vi "Ejemplo.vi"() -> ()   [LabVIEW 2020]
panel:
  in  "Tabla":string[][](table) caption="Result Set (from first statement with results)"
  in  "Multicolumn Listbox":i32(listbox)
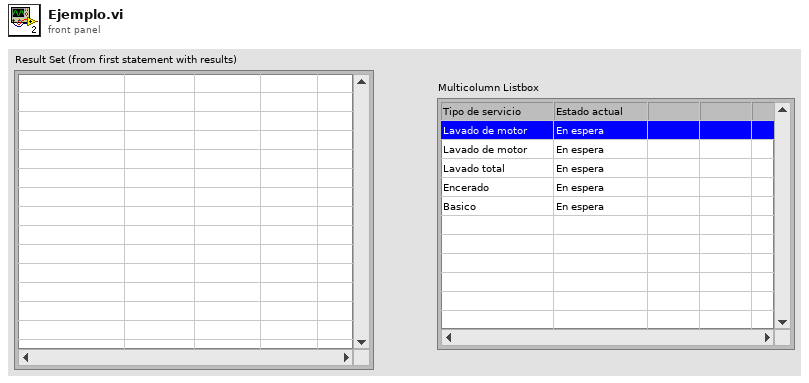
[diagram p1: front panel]
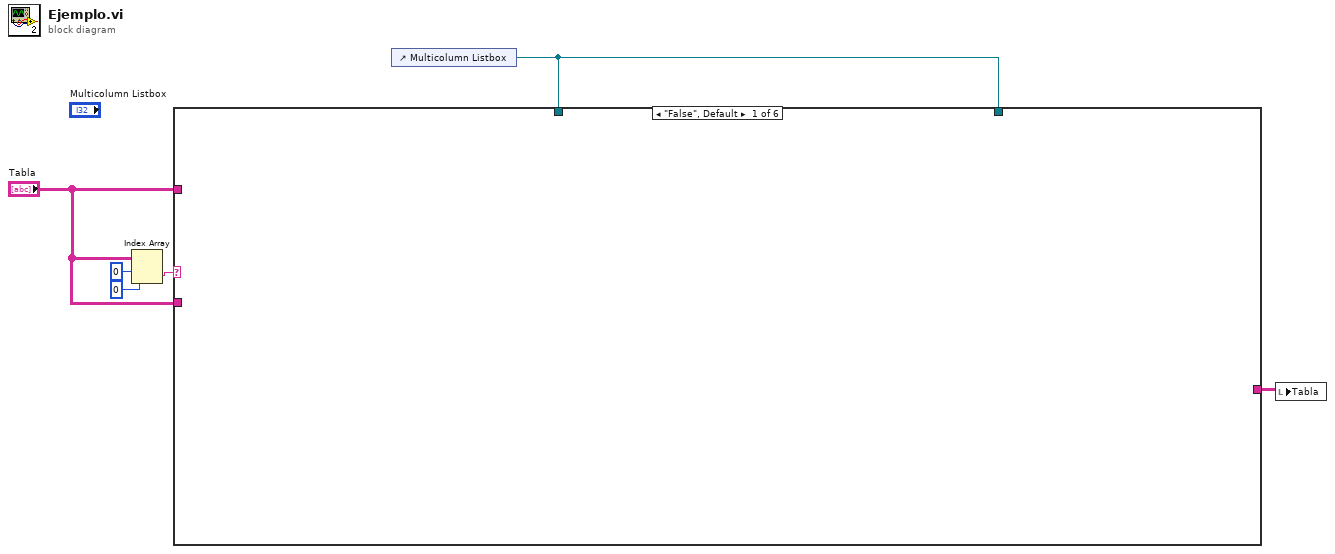
[diagram p0: block diagram]
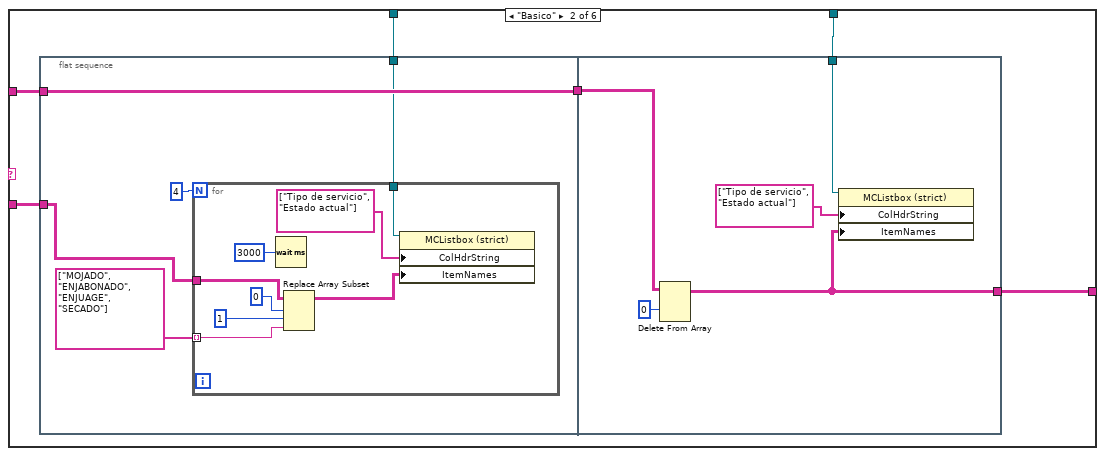
[diagram p2: hidden frame]
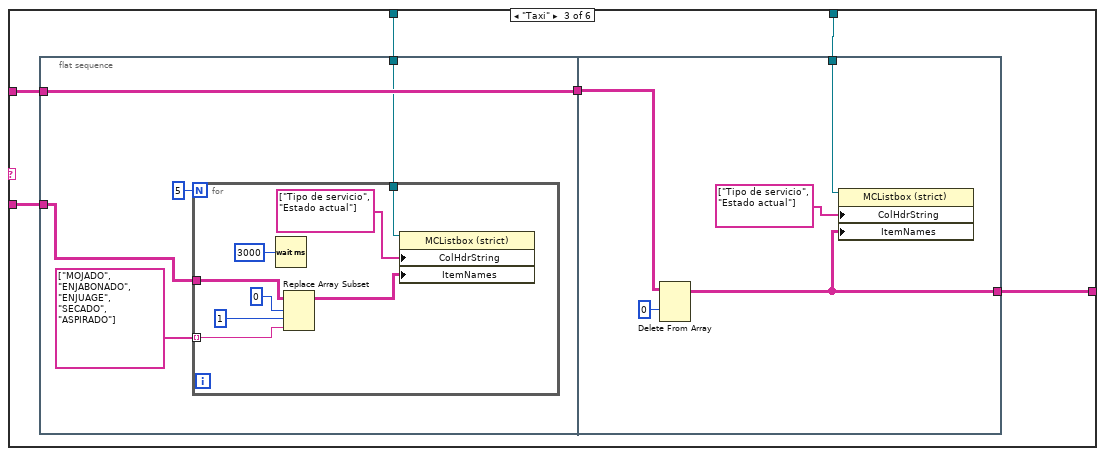
[diagram p3: hidden frame]
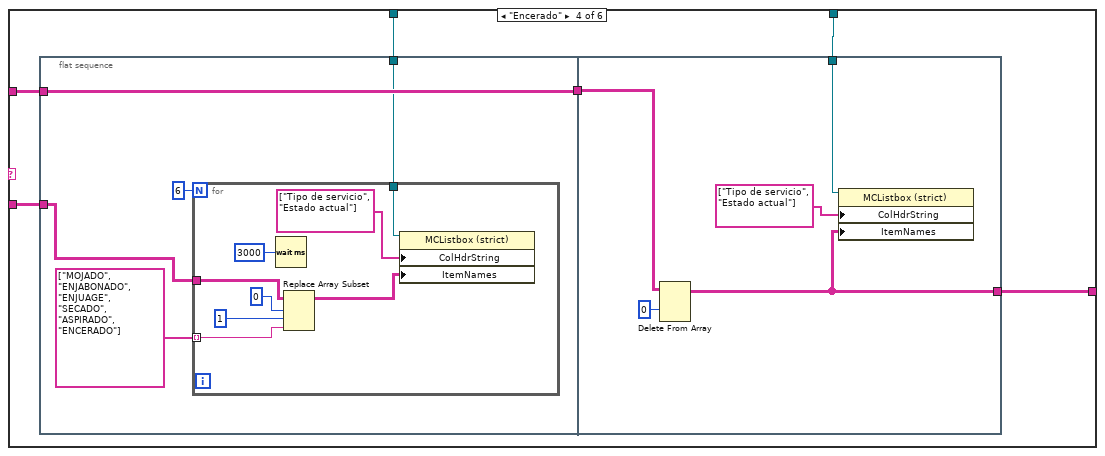
[diagram p4: hidden frame]
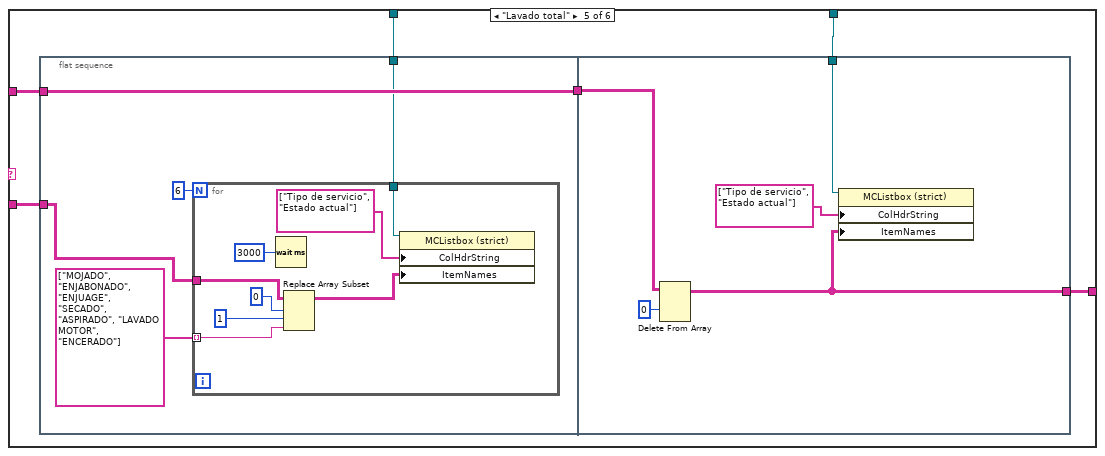
[diagram p5: hidden frame]
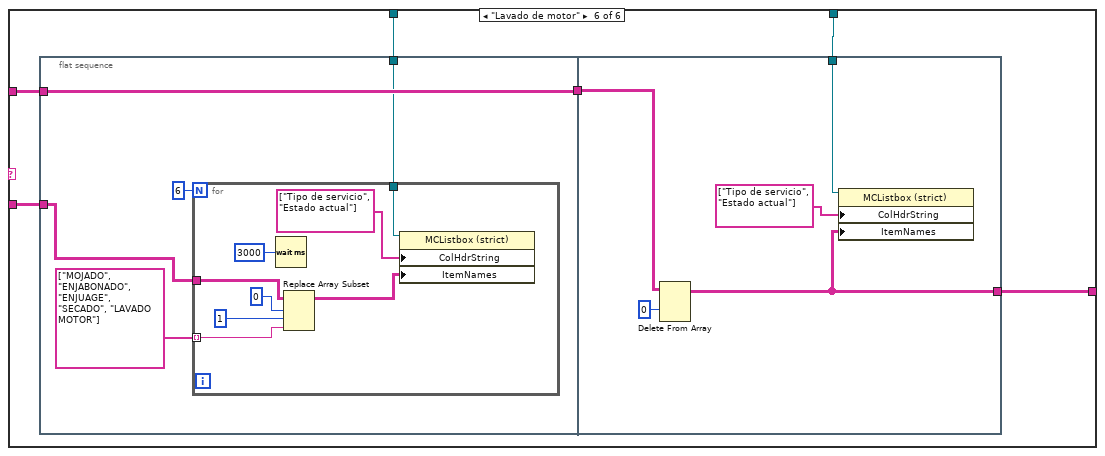
[diagram p6: hidden frame]
diagram:
  n1 = Index Array(array="Tabla", index (row)=0 ("index"), index (col)=0 ("disabled index (col)")) -> (element=w4:string)
  n2 = control-ref of="Multicolumn Listbox"() -> (w3:refnum<vi>)
  n3 = case shown="\"False\", Default" w4 {
    tunnel: "Tabla" -> [_ w12 w36 w60 w84 w108]
    tunnel: "Tabla" -> [_ w11 w35 w59 w83 w107]
    tunnel: w3 -> [_ w9 w33 w57 w81 w105]
    tunnel: w3 -> [_ w8 w32 w56 w80 w104]
    tunnel: [_ w7 w31 w55 w79 w103] -> w1
    frame "False", Default {
    }
    frame "Basico" {
      n4 = flat-sequence {
        tunnel: w12 -> [w15]
        tunnel: w11 -> [w14]
        tunnel: [w14] -> w10
        tunnel: w8 -> [w13]
        tunnel: w10 -> [w28]
        tunnel: w9 -> [w30]
        tunnel: [w26] -> w7
        frame #0 {
          n5 = for {
            N: 4 -> [_]
            tunnel: w15 -> [w25]
            tunnel: string[] ["MOJADO", "ENJABONADO", "ENJUAGE", "SECADO"] -> [w22] mode=indexing
            tunnel: w13 -> [w18]
            n6 = Wait (ms)(milliseconds to wait=u32 3000) -> ()  [unwired: 1 out]
            n7 = Replace Array Subset(array=w25, new element=w22, index (row)=0, index (col)=1 ("disabled index (col)")) -> (w19:string[][])
            n8 = property on="Property Node" class="MCListbox (strict)"(reference=w18, "ColHdrString"=string[] ["Tipo de servicio", "Estado actual"] ("Column Header Strings[]"), "ItemNames"=w19) -> ()  [unwired: 1 in, 2 out]
          }
        }
        frame #1 {
          n9 = Delete From Array(array=w28, index (row)=0) -> (array with subset deleted=w26:string[][])  [unwired: 2 in, 1 out]
          n10 = property on="Property Node" class="MCListbox (strict)"(reference=w30, "ColHdrString"=string[] ["Tipo de servicio", "Estado actual"] ("Column Header Strings[]"), "ItemNames"=w26) -> ()  [unwired: 1 in, 2 out]
        }
      }
    }
    frame "Taxi" {
      n11 = flat-sequence {
        tunnel: w36 -> [w39]
        tunnel: w35 -> [w38]
        tunnel: [w38] -> w34
        tunnel: w32 -> [w37]
        tunnel: w34 -> [w52]
        tunnel: w33 -> [w54]
        tunnel: [w50] -> w31
        frame #0 {
          n12 = for {
            N: 5 -> [_]
            tunnel: w39 -> [w49]
            tunnel: string[] ["MOJADO", "ENJABONADO", "ENJUAGE", "SECADO", "ASPIRADO"] -> [w46] mode=indexing
            tunnel: w37 -> [w42]
            n13 = Wait (ms)(milliseconds to wait=u32 3000) -> ()  [unwired: 1 out]
            n14 = Replace Array Subset(array=w49, new element=w46, index (row)=0, index (col)=1 ("disabled index (col)")) -> (w43:string[][])
            n15 = property on="Property Node" class="MCListbox (strict)"(reference=w42, "ColHdrString"=string[] ["Tipo de servicio", "Estado actual"] ("Column Header Strings[]"), "ItemNames"=w43) -> ()  [unwired: 1 in, 2 out]
          }
        }
        frame #1 {
          n16 = Delete From Array(array=w52, index (row)=0) -> (array with subset deleted=w50:string[][])  [unwired: 2 in, 1 out]
          n17 = property on="Property Node" class="MCListbox (strict)"(reference=w54, "ColHdrString"=string[] ["Tipo de servicio", "Estado actual"] ("Column Header Strings[]"), "ItemNames"=w50) -> ()  [unwired: 1 in, 2 out]
        }
      }
    }
    frame "Encerado" {
      n18 = flat-sequence {
        tunnel: w60 -> [w63]
        tunnel: w59 -> [w62]
        tunnel: [w62] -> w58
        tunnel: w56 -> [w61]
        tunnel: w58 -> [w76]
        tunnel: w57 -> [w78]
        tunnel: [w74] -> w55
        frame #0 {
          n19 = for {
            N: 6 -> [_]
            tunnel: w63 -> [w73]
            tunnel: string[] ["MOJADO", "ENJABONADO", "ENJUAGE", "SECADO", "ASPIRADO", "ENCERADO"] -> [w70] mode=indexing
            tunnel: w61 -> [w66]
            n20 = Wait (ms)(milliseconds to wait=u32 3000) -> ()  [unwired: 1 out]
            n21 = Replace Array Subset(array=w73, new element=w70, index (row)=0, index (col)=1 ("disabled index (col)")) -> (w67:string[][])
            n22 = property on="Property Node" class="MCListbox (strict)"(reference=w66, "ColHdrString"=string[] ["Tipo de servicio", "Estado actual"] ("Column Header Strings[]"), "ItemNames"=w67) -> ()  [unwired: 1 in, 2 out]
          }
        }
        frame #1 {
          n23 = Delete From Array(array=w76, index (row)=0) -> (array with subset deleted=w74:string[][])  [unwired: 2 in, 1 out]
          n24 = property on="Property Node" class="MCListbox (strict)"(reference=w78, "ColHdrString"=string[] ["Tipo de servicio", "Estado actual"] ("Column Header Strings[]"), "ItemNames"=w74) -> ()  [unwired: 1 in, 2 out]
        }
      }
    }
    frame "Lavado total" {
      n25 = flat-sequence {
        tunnel: w84 -> [w87]
        tunnel: w83 -> [w86]
        tunnel: [w86] -> w82
        tunnel: w80 -> [w85]
        tunnel: w82 -> [w100]
        tunnel: w81 -> [w102]
        tunnel: [w98] -> w79
        frame #0 {
          n26 = for {
            N: 6 -> [_]
            tunnel: w87 -> [w97]
            tunnel: string[] ["MOJADO", "ENJABONADO", "ENJUAGE", "SECADO", "ASPIRADO", "LAVADO MOTOR", "ENCERADO"] -> [w94] mode=indexing
            tunnel: w85 -> [w90]
            n27 = Wait (ms)(milliseconds to wait=u32 3000) -> ()  [unwired: 1 out]
            n28 = Replace Array Subset(array=w97, new element=w94, index (row)=0, index (col)=1 ("disabled index (col)")) -> (w91:string[][])
            n29 = property on="Property Node" class="MCListbox (strict)"(reference=w90, "ColHdrString"=string[] ["Tipo de servicio", "Estado actual"] ("Column Header Strings[]"), "ItemNames"=w91) -> ()  [unwired: 1 in, 2 out]
          }
        }
        frame #1 {
          n30 = Delete From Array(array=w100, index (row)=0) -> (array with subset deleted=w98:string[][])  [unwired: 2 in, 1 out]
          n31 = property on="Property Node" class="MCListbox (strict)"(reference=w102, "ColHdrString"=string[] ["Tipo de servicio", "Estado actual"] ("Column Header Strings[]"), "ItemNames"=w98) -> ()  [unwired: 1 in, 2 out]
        }
      }
    }
    frame "Lavado de motor" {
      n32 = flat-sequence {
        tunnel: w108 -> [w111]
        tunnel: w107 -> [w110]
        tunnel: [w110] -> w106
        tunnel: w104 -> [w109]
        tunnel: w106 -> [w124]
        tunnel: w105 -> [w126]
        tunnel: [w122] -> w103
        frame #0 {
          n33 = for {
            N: 6 -> [_]
            tunnel: w111 -> [w121]
            tunnel: string[] ["MOJADO", "ENJABONADO", "ENJUAGE", "SECADO", "LAVADO MOTOR"] -> [w118] mode=indexing
            tunnel: w109 -> [w114]
            n34 = Wait (ms)(milliseconds to wait=u32 3000) -> ()  [unwired: 1 out]
            n35 = Replace Array Subset(array=w121, new element=w118, index (row)=0, index (col)=1 ("disabled index (col)")) -> (w115:string[][])
            n36 = property on="Property Node" class="MCListbox (strict)"(reference=w114, "ColHdrString"=string[] ["Tipo de servicio", "Estado actual"] ("Column Header Strings[]"), "ItemNames"=w115) -> ()  [unwired: 1 in, 2 out]
          }
        }
        frame #1 {
          n37 = Delete From Array(array=w124, index (row)=0) -> (array with subset deleted=w122:string[][])  [unwired: 2 in, 1 out]
          n38 = property on="Property Node" class="MCListbox (strict)"(reference=w126, "ColHdrString"=string[] ["Tipo de servicio", "Estado actual"] ("Column Header Strings[]"), "ItemNames"=w122) -> ()  [unwired: 1 in, 2 out]
        }
      }
    }
  }
  n39 = local write "Tabla"(w1) -> ()
